vi "Color Sensor V3 CIE XYZ to Lab.vi"(7 "Illuminant (D65)":cluster{"Xn":dbl, "Yn":dbl, "Zn":dbl}={"Xn"=95.0489, "Yn"=100.0, "Zn"=108.884}, 11 "CIE XYZ":cluster{"X":dbl, "Y":dbl, "Z":dbl}) -> (2 "CIE Hue":dbl, 3 "CIE Lab":cluster{"L":dbl, "a":dbl, "b":dbl})   [LabVIEW 2023]
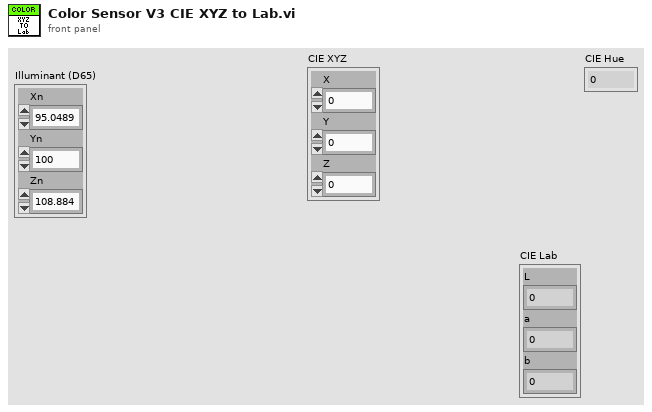
[diagram p1: front panel]
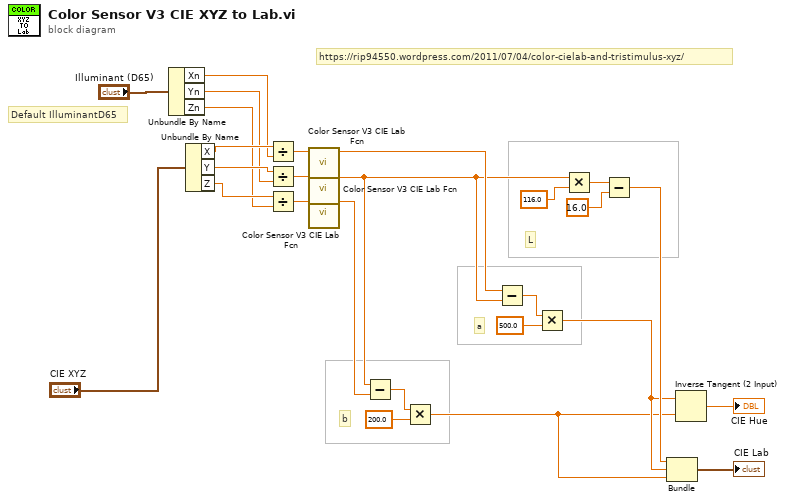
[diagram p0: block diagram]
diagram:
  # "b"
  # "a"
  # "https://rip94550.wordpress.com/2011/07/04/color-cielab-and-tristimulus-xyz/"
  # "L"
  # "Default IlluminantD65"
  n1 = Unbundle By Name("Illuminant (D65)") -> ("Xn"=w3:dbl, "Yn"=w2:dbl, "Zn"=w1:dbl)
  n2 = Unbundle By Name("CIE XYZ") -> ("X"=w25:dbl, "Y"=w24:dbl, "Z"=w23:dbl)
  n3 = Divide(x=w25, y=w3) -> (x/y=w20:dbl)
  n4 = Divide(x=w24, y=w2) -> (x/y=w19:dbl)
  n5 = Divide(x=w23, y=w1) -> (x/y=w18:dbl)
  n6 = call "Color Sensor V3 CIE Lab Fcn.vi"("x"=w20) -> ("y"=w12:dbl)  [unwired: 10 in]
  n7 = call "Color Sensor V3 CIE Lab Fcn.vi"("x"=w19) -> ("y"=w9:dbl)  [unwired: 10 in]
  n8 = call "Color Sensor V3 CIE Lab Fcn.vi"("x"=w18) -> ("y"=w8:dbl)  [unwired: 10 in]
  n9 = Subtract(x=w9, y=w8) -> (x-y=w11:dbl)
  n10 = Multiply(x=w11, y=200.0) -> (x*y=w6:dbl)
  n11 = Subtract(x=w12, y=w9) -> (x-y=w13:dbl)
  n12 = Multiply(x=w13, y=500.0) -> (x*y=w7:dbl)
  n13 = Multiply(x=w9, y=116.0) -> (x*y=w17:dbl)
  n14 = Subtract(x=w17, y=16.0) -> (x-y=w15:dbl)
  n15 = Bundle(w15, w7, w6) -> (→"CIE Lab":cluster{dbl, dbl, dbl})  [unwired: 1 in]
  n16 = Inverse Tangent (2 Input)(1:w6, 2:w7) -> (0:→"CIE Hue":dbl)
